vi "Flavour Descriptor.vi"(10 "Flavour":string, 11 "Descriptor":string) -> (3 "Flavoured Descriptor":string)   [LabVIEW 2015]
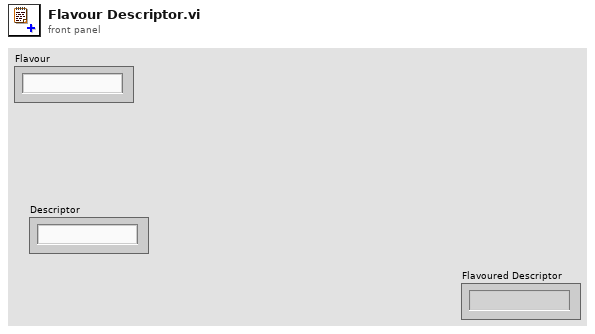
[diagram p1: front panel]
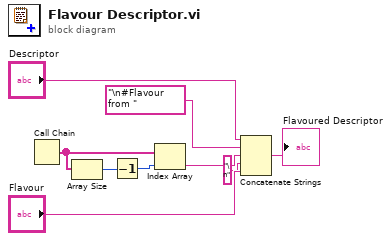
[diagram p0: block diagram]
diagram:
  n1 = Call Chain() -> (call chain=w7:string[])
  n2 = Array Size(array=w7) -> (size(s)=w6:i32)
  n3 = Decrement(x=w6) -> (x-1=w5:i32)
  n4 = Index Array(array=w7, index=w5) -> (element=w3:string)
  n5 = Concatenate Strings("Descriptor", "\n#Flavour from " ("string"), w3, "\n" ("string"), "Flavour") -> (→"Flavoured Descriptor":string)
